vi "RSA306 hi with FFTsub3.vi"() -> ()   [LabVIEW 2016]
doc: "This VI demonstrates a simple procedure for setting up a spectrum analyzer, running an acquisition, and retrieving and plotting the waveform data.\n\nString indicators Binary WF Data and Sgl Float WF Data are initialized to empty strings. Waveform Graph is initialized to 0 for 100000 locations (just an arbitrary number for demonstration purposes).\n\ntkrsa6100 Initialize.vi opens the VISA Resource Name from the information entered by the user. It also presets the instrument by default to the Spectrum measurement. On completion it passes dup VISA Resource Name and error out to the following drivers.\n\nThe next VI to execute is tkrsa6100 Config Frequency.vi. Numeric control Center Freq (MHz)(50) is passed to the VI to set the center frequency to the default 50MHz value. The Set/Read Freq Setting (Set) is not wired since it defaults to SET, which is what is desired in this case. This is the case for all the configuration VI's in the example.\n\nThe next VI to execute is tkrsa6100 Config Spectrum Settings.vi. Enumerated control Spectrum Settings (CENTER FREQUENCY) is passed a Frequency Span constant and numeric control Freq Span (MHz) (40) to set the span to 40MHz.\n\nNext the reference level is set using tkrsa6100 Config RF Input.vi. Enumerated control Input Setting (REFERENCE LEVEL) is passed a Reference Level constant and numeric control Ref Level (dBm)(0) to set the reference level to 0dBm.\n\nNext the acquisition mode is set to single acquisition using tkrsa6100 Config Acquisition.vi. No parameters are passed since the default setting of this VI sets the acquisition mode to single.\n\nA single acquisition is then performed using tkrsa6100 Run Single Acquisition.vi. This VI sends an INIT command followed by a *OPC? Query. When the acquisition is completed the instrument returns a 1 and the next vi executes.\n\nThe binary waveform data is then retrieved by tkrsa6100 Spectrum Msmt Results.vi. The last acquisition data is retrieved by passing constant GET LAST ACQUISITION RESULT to enumerated input Run Acquisition and/or Get Result (RUN ACQUISITION & GET RESULT). The binary data is converted to a comma separated list of single precision floating point numbers by passing constant YES to enumerated input Convert Resp String (NO). The number of display points (total number of data bytes/4) is passed to a Spectral Display property node to scale the x axis of the graph. The binary data string from output Measurement Response String is copied to string indicator Binary WF Data. The converted binary data from output Converted Sgl Float Response String is copied to string indicator Sgl Float WF Data.\n\nSgl Float WF Data is then converted to an array by function Spreadsheet String to Array using a comma as the data separator. The output array is then passed to waveform graph Spectral Display for viewing.\n\nThe VISA Resource Name is closed using tkrsa6100 Close.vi."
uses:
  <vilib>/Analysis/baseanly.llb/Mean (DBL).vi
  <vilib>/Analysis/NI_AALBase.lvlib
panel:
  out "Peak vs time":cluster{i32[], dbl[]}(graph)
  out "mean":dbl format="%0.2f"
  out "Amp in range":dbl[](array[numeric])
  out "Pts in range":dbl[](array[numeric])
  in  "Marker Freq stop":dbl
  out "fractional index or x":dbl
  in  "Marker Freq start":dbl
  in  "stop 2":bool
  in  "RSA Control Cluster":T1={"Center Freq (MHz)"=20.0, "Freq Span (MHz)"=20.0, "Ref Level (dBm)"=0.0, "# Points"=enum."801", "Analysis Length (ms)"=0.022, "Trigger Settings\n(TRIGGER SOURCE)"=enum."TRIGGER ON"} {"Analysis Length (ms)" step=1e-09; "Ref Level (dBm)" min=-170.0 max=50.0 step=0.1}
  out "Metrics:Total Data Size":u32
  out "Metrics:Size of Front Panel":u32
  out "Freq Out Cluster":T2
  out "cursor diff":dbl
  out "iteration":i32
  out "# of Pts Between Cursors":dbl
  out "Cursor 1 X":dbl
  out "Cursor 0 X":dbl
  out "I & Q full":cluster{dbl[], "I or Q Data Array":sgl[]}[](graph)
  out "# of Spectrum pts retrieved":i32
  in  "stop":bool=TRUE
  in  "beta":dbl format="%0.2f"
  in  "Use windowing":bool
  out "FFT out From RSA":cluster{dbl[], "FFT {X}":dbl[]}(graph)
  out "FFT^2 from I&Q":cluster{dbl[], "FFT {X}":dbl[]}(graph)={[72.99999907342773, 73.14432898943954, 73.28865890545134, 73.43298882146314, 73.57731873747494, 73.72164865348674, 73.86597856949854, 74.01030848551034, 74.15463840152213, 74.29896831753393, 74.44329823354573, 74.58762814955753, 74.73195806556933, 74.87628798158114, 75.02061789759293, 75.16494781360473, 75.30927772961653, 75.45360764562834, 75.59793756164012, 75.74226747765192, 75.88659739366372, 76.03092730967553, 76.17525722568732, 76.31958714169912, 76.46391705771092, 76.60824697372273, 76.75257688973453, 76.89690680574631, 77.04123672175811, 77.18556663776992, 77.32989655378172, 77.4742264697935, 77.6185563858053, 77.76288630181712, 77.90721621782892, 78.05154613384072, 78.1958760498525, 78.34020596586431, 78.48453588187611, 78.62886579788791, 78.7731957138997, 78.91752562991151, 79.06185554592331, 79.2061854619351, 79.35051537794689, 79.4948452939587, 79.6391752099705, 79.7835051259823, 79.9278350419941, 80.0721649580059, 80.2164948740177, 80.3608247900295, 80.5051547060413, 80.64948462205311, 80.7938145380649, 80.93814445407669, 81.08247437008849, 81.2268042861003, 81.37113420211209, 81.51546411812389, 81.65979403413569, 81.8041239501475, 81.94845386615928, 82.09278378217108, 82.23711369818288, 82.3814436141947, 82.5257735302065, 82.67010344621828, 82.81443336223008, 82.95876327824189, 83.10309319425369, 83.24742311026547, 83.39175302627727, 83.53608294228908, 83.68041285830088, 83.82474277431268, 83.96907269032447, 84.11340260633628, 84.25773252234808, 84.40206243835988, 84.54639235437166, 84.69072227038347, 84.83505218639527, 84.97938210240707, 85.12371201841886, 85.26804193443067, 85.41237185044247, 85.55670176645427, 85.70103168246607, 85.84536159847787, 85.98969151448966, 86.13402143050146, 86.27835134651326, 86.42268126252506, 86.56701117853686, 86.71134109454866, 86.85567101056046], "FFT {X}"=[2.273932630988823e-07, 1.1331146319928143e-07, 7.673719462960696e-08, 4.8490746468829755e-06, 1.6442867833395572e-06, 3.16436268703382e-06, 2.639540533574584e-06, 3.334839091433884e-06, 4.600463519168855e-07, 7.66410378536425e-06, 2.1359108019339082e-05, 3.163756375846005e-05, 1.7486392953015998e-06, 5.819774956187226e-05, 1.7641054577208325e-05, 1.6979948996099875e-05, 6.2693899532632095e-06, 2.3345502675972444e-06, 3.1376219779214914e-05, 2.03224790497132e-05, 1.615880551905034e-05, 1.0387525314792172e-05, 1.5288981152198085e-05, 8.951089675188266e-05, 5.220838568835042e-06, 3.951059482528036e-06, 2.2455332453227875e-05, 4.043265080177603e-05, 1.3603674976209462e-05, 1.4610779340262739e-05, 6.778155093094428e-06, 5.92310092221894e-05, 0.00012371060242161107, 4.2293965227730726e-05, 4.793949807803902e-06, 1.703774948817084e-05, 4.1046539738076146e-05, 1.0575250111078698e-05, 1.5838772387061695e-05, 5.963059605451412e-06, 8.322466613350297e-06, 4.241894423745356e-05, 2.5902944249513385e-05, 3.754440849478757e-06, 2.2684130780756104e-06, 1.4792708956558557e-06, 2.8052728218109083e-06, 9.519822607230608e-06, 2.5898912044999134e-07, 1.5674000233301835e-05, 1.3652167200969293e-06, 1.9463849822553144e-06, 3.654050359843304e-05, 1.1291499237591179e-05, 6.364356455835304e-06, 1.5162644733310776e-05, 2.498743892235212e-05, 2.59215466998731e-05, 2.5356348978855883e-05, 3.372928674635838e-05, 3.2302722433788863e-06, 6.456706467716242e-06, 1.458542775043343e-05, 6.265393201875059e-06, 1.0526946272506417e-05, 1.3629572719674517e-05, 5.08190028344042e-06, 8.753167304918669e-06, 1.0618177493791915e-05, 4.256799122932561e-05, 6.634457042403187e-06, 1.2110046839534622e-05, 3.4087842403903063e-06, 6.274698806587281e-06, 1.7395492102973268e-05, 6.128606933081257e-05, 8.034267247831298e-05, 2.2934113274395202e-05, 3.215895946795535e-05, 1.0317162977800269e-06, 2.8731735651279777e-07, 2.8598897809844725e-05, 1.773915488316907e-06, 2.4559181515814637e-05, 6.51682013725626e-05, 1.3429668418120791e-05, 1.5195877753597404e-05, 7.288765358591678e-06, 1.8987776629762155e-05, 2.3445741553836735e-05, 2.5513476948437664e-06, 7.888513041438307e-07, 1.3567788998363706e-06, 2.0658168696090098e-06, 5.785587479331871e-07, 2.8232882934250476e-07, 2.6643643406101695e-07]}
  out "FreqStep":dbl
  out "I & Q  partial":cluster{dbl[], sgl[]}[](graph)
  out "# I or Q Pts":i32
  in  "VISA Resource Name":refnum<visa-resource-name>="TCPIP0::127.0.0.1::inst0::INSTR"
  out "Sgl Float WF Data":string
  out "Binary WF Data":string
  out "Spectral Display":dbl[](graph)=[-100.550338745117, -100.865898132324, -100.055114746094, -100.513687133789, -98.912384033203, -101.86759185791, -99.886054992676, -98.280754089355, -99.356986999512, -99.41291809082, -100.67155456543, -100.569961547852, -101.467147827148, -99.184501647949, -101.941261291504, -100.212478637695, -101.129829406738, -100.52604675293, -100.7939453125, -100.198677062988, -100.002563476562, -101.958740234375, -99.303619384766, -98.484771728516, -100.796211242676, -101.325035095215, -101.804656982422, -100.850593566895, -101.298637390137, -99.770805358887, -98.808280944824, -101.318023681641, -99.57886505127, -100.508224487305, -100.616767883301, -100.600654602051, -99.123565673828, -101.568901062012, -98.457931518555, -99.805709838867, -99.298568725586, -102.226028442383, -100.700386047363, -99.445762634277, -100.692687988281, -100.283546447754, -101.525848388672, -101.59400177002, -100.571098327637, -100.408309936523, -101.573852539062, -100.876373291016, -99.473991394043, -98.885787963867, -99.478179931641, -99.414611816406, -100.745628356934, -100.405769348145, -100.550086975098, -101.737022399902, -100.464469909668, -102.024978637695, -100.643768310547, -100.495559692383, -100.85823059082, -100.459129333496, -100.412284851074, -99.047401428223, -100.545104980469, -100.606239318848, -100.008010864258, -101.58097076416, -99.201164245605, -100.060760498047, -99.007080078125, -98.575668334961, -100.801124572754, -101.846046447754, -100.409858703613, -99.658515930176, -87.074851989746, -101.954887390137, -101.25106048584, -100.35228729248, -100.468887329102, -100.489883422852, -100.308792114258, -99.900894165039, -100.278121948242, -99.058067321777, -99.013816833496, -100.399383544922, -101.039794921875, -98.751235961914, -101.476287841797, -100.809410095215, -101.54175567627, -100.014114379883, -98.903923034668, -100.957069396973, -100.160820007324, -100.303314208984, -101.395530700684, -101.13591003418, -100.250480651855, -100.815155029297, -101.235824584961, -100.353385925293, -100.524604797363, -101.694984436035, -100.57209777832, -100.20694732666, -100.339385986328, -100.5029296875, -102.065803527832, -100.840377807617, -101.361434936523, -102.486083984375, -99.822219848633, -99.708770751953, -100.815650939941, -99.921195983887, -99.004348754883, -101.069366455078, -100.102096557617, -101.359786987305, -100.169326782227, -100.855087280273, -100.436889648437, -99.430320739746, -102.201194763184, -98.398323059082, -100.264114379883, -101.190093994141, -97.551864624023, -99.804649353027, -100.999176025391, -102.163314819336, -99.233787536621, -101.160591125488, -102.859664916992, -100.933372497559, -99.543952941895, -101.640991210937, -100.737907409668, -100.88272857666, -99.914588928223, -100.99201965332, -99.82975769043, -99.958145141602, -100.332321166992, -99.202865600586, -98.971542358398, -101.199119567871, -100.002639770508, -100.379287719727, -102.733993530273, -101.047821044922, -101.062637329102, -100.490631103516, -99.570091247559, -100.822036743164, -99.495933532715, -99.691299438477, -101.119491577148, -99.969169616699, -101.370628356934, -101.276794433594, -100.304641723633, -97.739120483398, -99.724952697754, -98.052604675293, -101.780364990234, -99.872802734375, -101.446601867676, -100.011825561523, -100.626129150391, -100.016258239746, -100.463325500488, -100.814552307129, -98.368011474609, -101.450942993164, -98.984527587891, -99.13134765625, -101.283500671387, -101.268920898437, -99.028633117676, -99.825736999512, -99.720832824707, -101.301513671875, -101.047241210937, -100.3115234375, -100.123146057129, -99.407669067383, -99.631744384766, -100.10962677002, -100.001708984375, -102.515518188477, -98.70344543457, -100.51188659668, -98.830825805664, -99.284408569336, -100.024505615234, -98.385818481445, -100.892181396484, -99.685241699219, -98.992698669434, -99.39395904541, -100.281867980957, -99.531661987305, -100.906555175781, -99.699020385742, -100.121429443359, -98.757469177246, -99.419845581055, -97.976013183594, -101.205871582031, -100.501953125, -100.021583557129, -100.356979370117, -100.71753692627, -100.46329498291, -100.892501831055, -101.838409423828, -101.372383117676, -99.252029418945, -99.76936340332, -98.654335021973, -100.489685058594, -99.062408447266, -101.665840148926, -99.905433654785, -101.712501525879, -99.85466003418, -100.939422607422, -98.979385375977, -101.255149841309, -101.09969329834, -100.925674438477, -100.328742980957, -99.538612365723, -98.808433532715, -100.842529296875, -100.238067626953, -101.345428466797, -100.050537109375, -100.399284362793, -100.017051696777, -99.849670410156, -100.567657470703, -100.343772888184, -99.282569885254, -100.663917541504, -101.199584960937, -101.901153564453, -101.351409912109, -98.658866882324, -99.848770141602, -101.877182006836, -100.49617767334, -101.537330627441, -100.924682617187, -97.984771728516, -100.308158874512, -100.322402954102, -100.767883300781, -100.310073852539, -100.786071777344, -101.351623535156, -100.523536682129, -101.092514038086, -100.754669189453, -99.298774719238, -100.813056945801, -99.991065979004, -101.504623413086, -101.232765197754, -100.107154846191, -99.418594360352, -98.61107635498, -99.415710449219, -101.472129821777, -100.912246704102, -99.791061401367, -101.327758789062, -100.108337402344, -100.526657104492, -99.587135314941, -98.377944946289, -100.356819152832, -99.85327911377, -100.841262817383, -98.974731445312, -99.606948852539, -102.143646240234, -98.766189575195, -99.99284362793, -100.895263671875, -99.367050170898, -99.253242492676, -100.08667755127, -100.553131103516, -100.857391357422, -101.711227416992, -99.825546264648, -98.692436218262, -99.648223876953, -99.844596862793, -99.068862915039, -101.533081054687, -99.982055664062, -100.804931640625, -96.95915222168, -100.675964355469, -100.574676513672, -99.792411804199, -100.516044616699, -99.432067871094, -101.020401000977, -100.661483764648, -101.725570678711, -99.595375061035, -100.06787109375, -99.804389953613, -102.322189331055, -98.901550292969, -101.507293701172, -99.793487548828, -100.540351867676, -100.780242919922, -100.127319335937, -100.003524780273, -99.602500915527, -98.637382507324, -101.011360168457, -99.077499389648, -100.247482299805, -97.887725830078, -102.085151672363, -99.34139251709, -100.531723022461, -100.816795349121, -102.088920593262, -100.546455383301, -102.192306518555, -99.071624755859, -100.28343963623, -100.598419189453, -99.334259033203, -99.664779663086, -97.886917114258, -99.813995361328, -100.696228027344, -101.955505371094, -102.258979797363, -102.029754638672, -100.8662109375, -100.926208496094, -100.807052612305, -101.128890991211, -98.354034423828, -99.024314880371, -101.485443115234, -101.602096557617, -97.892822265625, -101.470703125, -98.830749511719, -100.045959472656, -100.344650268555, -101.595001220703, -97.871208190918, -101.413185119629, -100.882888793945, -98.795585632324, -101.501831054687, -100.533180236816, -101.440567016602, -99.224174499512, -99.32649230957, -100.897682189941, -99.851852416992, -99.728507995605, -99.662971496582, -98.721755981445, -101.032135009766, -100.706283569336, -100.466918945312, -99.798248291016, -100.419586181641, -100.837371826172, -101.374435424805, -100.814964294434, -99.004135131836, -101.148536682129, -100.68058013916, -100.756843566895, -100.15885925293, -99.221481323242, -99.54581451416, -100.453453063965, -100.57795715332, -101.148979187012, -100.433052062988, -101.978225708008, -99.846565246582, -100.104637145996, -100.098175048828, -102.141723632812, -101.605690002441, -99.873359680176, -101.258079528809, -101.42431640625, -99.871452331543, -102.639274597168, -100.601585388184, -101.972610473633, -101.68872833252, -100.650726318359, -100.978286743164, -100.009384155273, -99.023010253906, -102.653121948242, -100.426239013672, -100.945854187012, -100.945205688477, -101.281471252441, -99.653778076172, -101.798393249512, -101.911247253418, -99.407638549805, -100.486267089844, -100.227569580078, -100.53246307373, -100.187919616699, -100.094390869141, -100.00910949707, -99.580986022949, -101.552139282227, -99.501281738281, -100.229248046875, -100.41072845459, -99.136566162109, -100.057098388672, -99.654800415039, -101.470153808594, -100.272033691406, -102.090690612793, -100.150230407715, -100.233016967773, -99.821128845215, -101.96110534668, -100.44783782959, -100.379745483398, -100.564086914062, -100.66283416748, -100.941314697266, -99.063705444336, -101.046104431152, -101.203369140625, -101.31706237793, -99.69482421875, -99.850654602051, -100.772903442383, -100.658180236816, -100.794387817383, -101.259185791016, -99.263107299805, -102.132049560547, -101.211318969727, -101.490661621094, -100.15983581543, -100.298202514648, -100.612930297852, -100.09033203125, -97.22306060791, -99.894561767578, -101.341903686523, -99.349258422852, -100.165794372559, -101.825523376465, -99.893409729004, -100.450881958008, -100.050659179687, -101.527481079102, -101.331695556641, -100.468971252441, -101.455322265625, -99.166534423828, -99.911262512207, -101.425621032715, -100.859977722168, -100.757179260254, -101.168304443359, -99.792510986328, -99.813842773437, -100.985527038574, -100.48152923584, -101.116722106934, -100.52799987793, -102.19359588623, -98.876556396484, -101.040328979492, -102.055938720703, -101.163955688477, -99.716537475586, -100.167327880859, -100.142478942871, -101.779495239258, -100.689811706543, -98.207588195801, -100.404693603516, -100.201606750488, -100.779479980469, -99.916084289551, -99.407791137695, -100.122749328613, -101.812606811523, -101.024642944336, -102.179672241211, -100.940444946289, -100.357330322266, -100.155799865723, -99.45484161377, -100.356147766113, -99.973617553711, -99.72966003418, -100.918563842773, -99.232574462891, -100.032485961914, -100.875595092773, -101.141540527344, -102.283218383789, -101.503074645996, -102.207214355469, -101.424591064453, -99.745712280273, -101.473587036133, -100.337684631348, -102.04655456543, -101.569664001465, -100.722312927246, -101.008522033691, -100.684356689453, -101.044158935547, -100.232864379883, -100.195053100586, -100.292091369629, -102.663642883301, -98.514129638672, -100.355270385742, -100.902053833008, -100.774368286133, -99.509002685547, -101.305000305176, -99.386489868164, -99.192878723145, -99.583618164062, -98.280197143555, -101.662719726562, -101.981384277344, -99.561195373535, -101.218673706055, -101.522567749023, -100.710975646973, -99.873352050781, -100.043991088867, -100.786987304687, -100.88207244873, -101.670349121094, -101.070434570312, -102.330474853516, -101.139305114746, -100.553726196289, -101.080917358398, -100.014381408691, -100.74267578125, -101.376068115234, -99.508666992187, -100.402755737305, -101.458442687988, -99.817077636719, -99.497161865234, -99.722450256348, -101.075325012207, -101.166007995605, -101.071212768555, -99.873245239258, -100.388832092285, -101.41625213623, -100.525978088379, -100.986129760742, -99.89119720459, -100.209266662598, -101.846252441406, -100.338325500488, -99.660354614258, -99.571578979492, -102.133171081543, -100.463859558105, -100.218765258789, -100.48420715332, -98.158195495605, -101.068511962891, -100.645751953125, -100.28645324707, -100.960067749023, -102.125846862793, -99.240020751953, -100.359405517578, -100.035057067871, -100.114097595215, -101.306259155273, -99.285079956055, -100.391830444336, -99.01554107666, -100.258865356445, -98.728218078613, -100.905616760254, -101.235694885254, -99.772598266602, -102.705078125, -99.118644714355, -100.937576293945, -99.03776550293, -100.502166748047, -100.544166564941, -100.152221679687, -99.755935668945, -101.306137084961, -101.620468139648, -100.771682739258, -97.545074462891, -99.748275756836, -99.849456787109, -99.425132751465, -101.4501953125, -100.094604492187, -101.045394897461, -100.365760803223, -100.378326416016, -99.960372924805, -99.518020629883, -98.761451721191, -100.071517944336, -99.611015319824, -100.961112976074, -99.728225708008, -101.468490600586, -100.286552429199, -100.593269348145, -100.339752197266, -100.324165344238, -100.608863830566, -100.953826904297, -102.148063659668, -100.073135375977, -101.460403442383, -100.869049072266, -100.91569519043, -99.907760620117, -100.546600341797, -99.498947143555, -98.508110046387, -101.926765441895, -97.669898986816, -99.041915893555, -100.350219726562, -99.40697479248, -100.568992614746, -101.795227050781, -100.295150756836, -100.469528198242, -100.674736022949, -101.288589477539, -100.309440612793, -101.232971191406, -97.823684692383, -101.273803710937, -101.031936645508, -100.720474243164, -101.440956115723, -100.856010437012, -98.955215454102, -101.424751281738, -99.771881103516, -101.40625, -101.204063415527, -101.750625610352, -100.588256835937, -102.470924377441, -101.291969299316, -101.423835754395, -98.857757568359, -102.00910949707, -100.523918151855, -100.347198486328, -100.93798828125, -101.508415222168, -100.711967468262, -99.973365783691, -99.873085021973, -100.742347717285, -100.09001159668, -100.524185180664, -101.417045593262, -101.220520019531, -102.689018249512, -102.225723266602, -101.284866333008, -100.547622680664, -101.23991394043, -102.037322998047, -100.880744934082, -100.685493469238, -100.668258666992, -100.301788330078, -99.016708374023, -102.30345916748, -99.447540283203, -100.94401550293, -86.783302307129, -100.292877197266, -101.487869262695, -100.213653564453, -102.028007507324, -98.812118530273, -100.086151123047, -101.277923583984, -101.078903198242, -100.103454589844, -98.755073547363, -101.702529907227, -99.214538574219, -98.939552307129, -100.480224609375, -98.694679260254, -99.073760986328, -100.033782958984, -101.073501586914, -100.257873535156, -99.690689086914, -100.311141967773, -102.31135559082, -101.017456054687, -99.194183349609, -100.42781829834, -102.232551574707, -100.907676696777, -98.880035400391, -100.672286987305, -101.721580505371, -100.515151977539, -98.296730041504, -101.345634460449, -99.50260925293, -100.800369262695, -99.824249267578, -101.611465454102, -97.455688476562, -102.069770812988, -100.366958618164, -100.448394775391, -99.052459716797, -98.817855834961, -101.656845092773, -99.100914001465, -101.839515686035, -101.317642211914, -100.746368408203, -99.396423339844, -100.516006469727, -102.368705749512, -99.86840057373, -101.438186645508, -100.931861877441, -101.522415161133, -99.652969360352, -101.873107910156, -99.384582519531, -100.033912658691, -99.868743896484, -101.091194152832, -101.110298156738, -100.822662353516, -99.58659362793, -100.84928894043, -100.407035827637, -100.647857666016, -98.793746948242, -100.717239379883, -101.495048522949, -102.786880493164, -101.375053405762, -101.189392089844, -101.156097412109, -100.519378662109, -102.34831237793, -100.975868225098, -100.173492431641, -99.891387939453, -100.191482543945]
  out "error out":errorcluster {"code" format="%#.0f"}
  # "This VI has the setup parameters entered in a sub VI\nThe FFT calculation is done in a loop that allows the # of pts\nto FFT to be selected. Also windowing can be changed.\nWhen happy about the FFT then push the STOP button.\nVersion just h is this VI before the setup sub VI was used"
  # "RSA306 Acquire and Fetch"
  # "Spectrum"
  # "Needs trigger input to work"
  # "IQ vs Time"
  # "To Do: Use these cursers to graphically select \nthe time window to FFT"
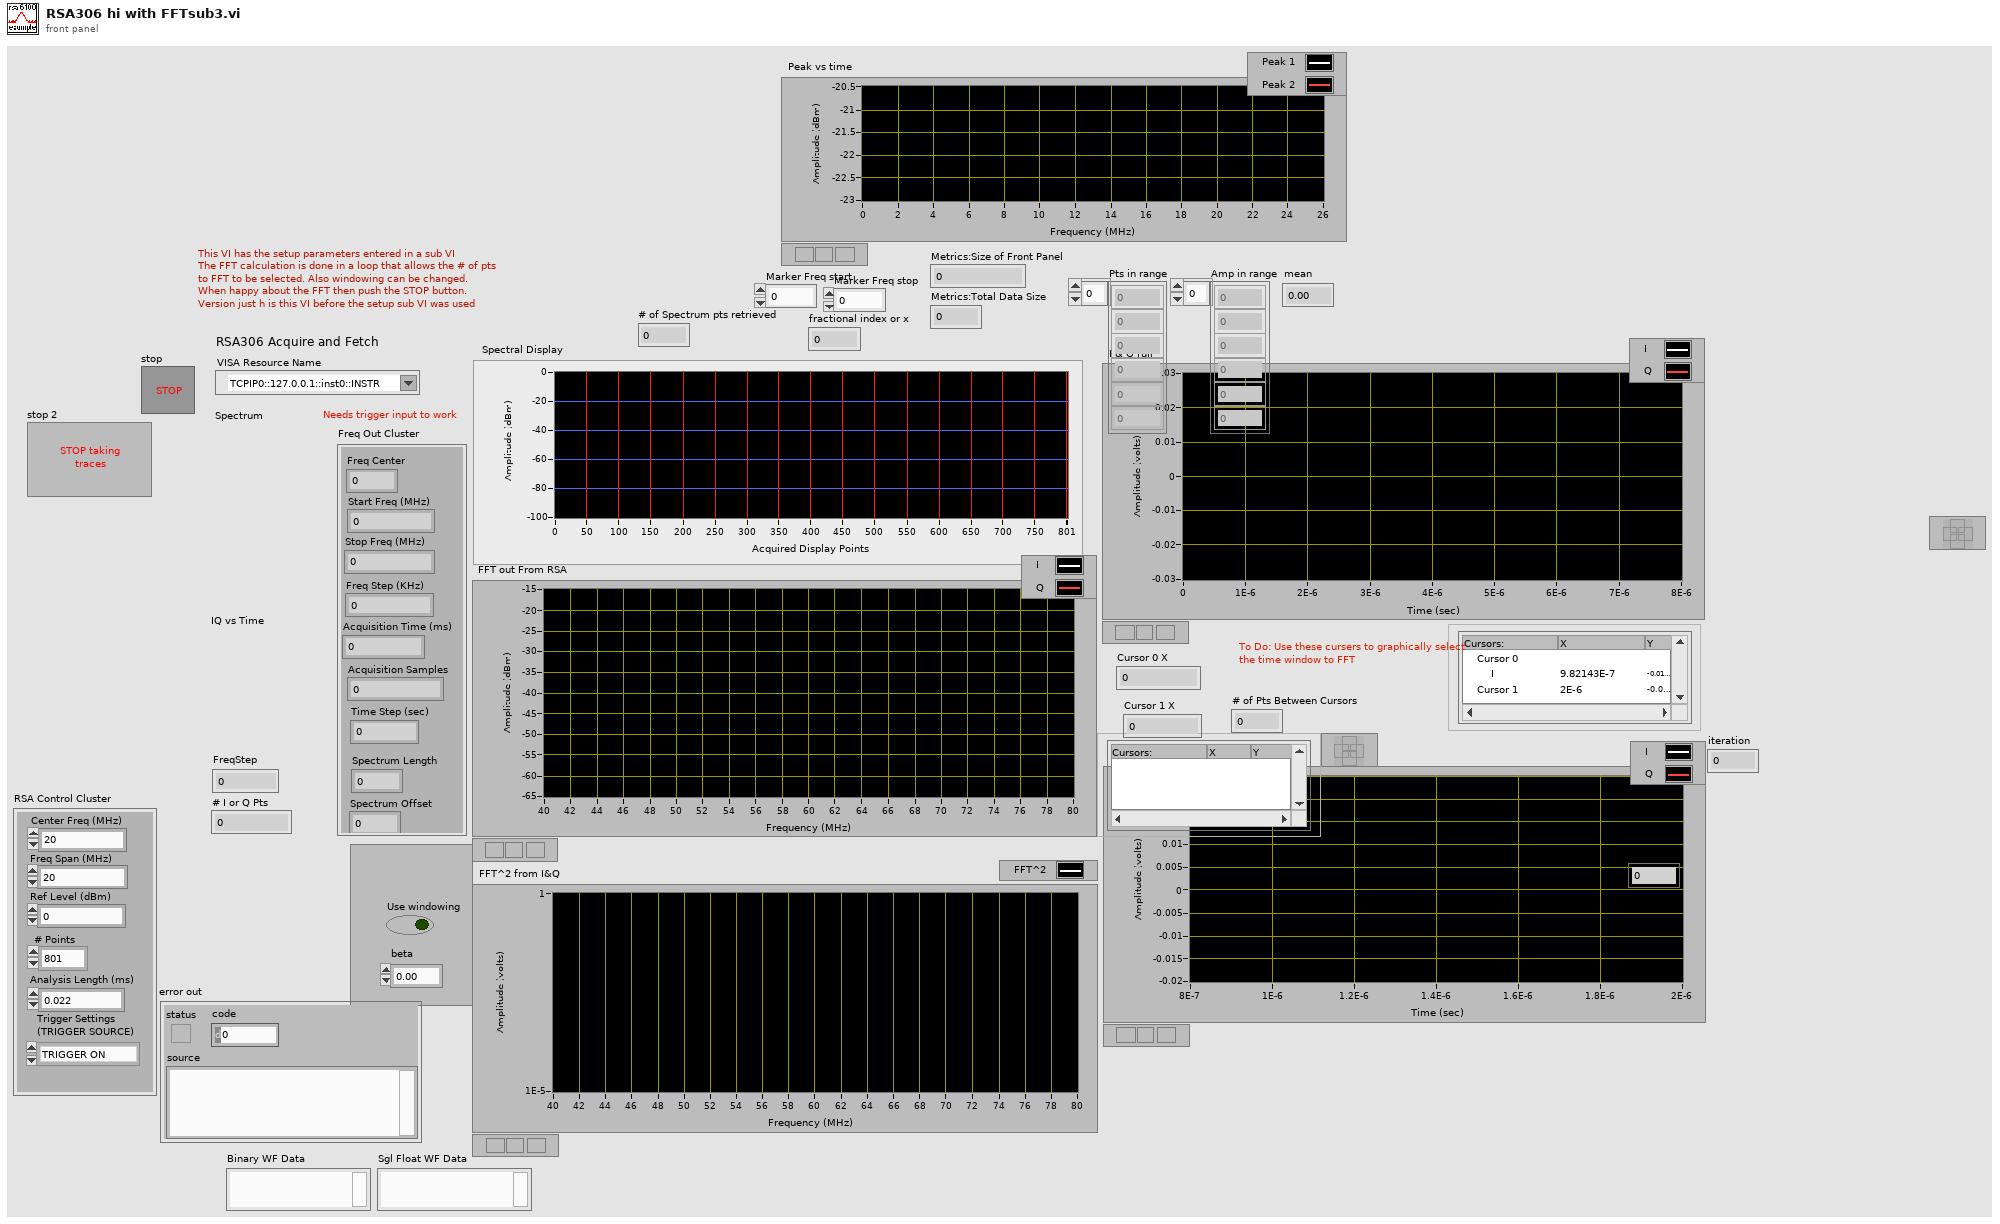
[diagram p1: front panel]
types:
  T1 = cluster{"Center Freq (MHz)":dbl, "Freq Span (MHz)":dbl, "Ref Level (dBm)":dbl, "# Points":enum16{"801", "2401", "4001", "8001", "10401", "16001", "32001", "64001"}, "Analysis Length (ms)":dbl, "Trigger Settings\n(TRIGGER SOURCE)":enum16{"TRIGGER SOURCE", "TRIGGER ON", "TRIGGER OFF", "TIME DELAY", "TIME POSITION", "TRIGGER EACH SEGMENT ON", "TRIGGER EACH SEGMENT OFF", "TRIGGER HOLDOFF ON", "TRIGGER HOLDOFF OFF", "TRIGGER HOLDOFF TIME", "FRONT EXT  LEVEL", "FRONT EXT IMPEDANCE", "FRONT EXT SLOPE", "REAR EXT SLOPE", "GATED TRIG2 (REAR) LOGIC", "FORCE TRIGGER (SET)"}}
  T2 = cluster{"Start Freq (MHz)":dbl, "Stop Freq (MHz)":dbl, "Freq Center":dbl, "Freq Step (KHz)":dbl, "Acquisition Time (ms)":dbl, "Acquisition Samples":dbl, "Time Step (sec)":dbl, "Spectrum Length":dbl, "Spectrum Offset":dbl}
  T3 = enum16{"RUN ACQUISITION  & GET RESULT", "GET LAST ACQUISITION RESULT"}
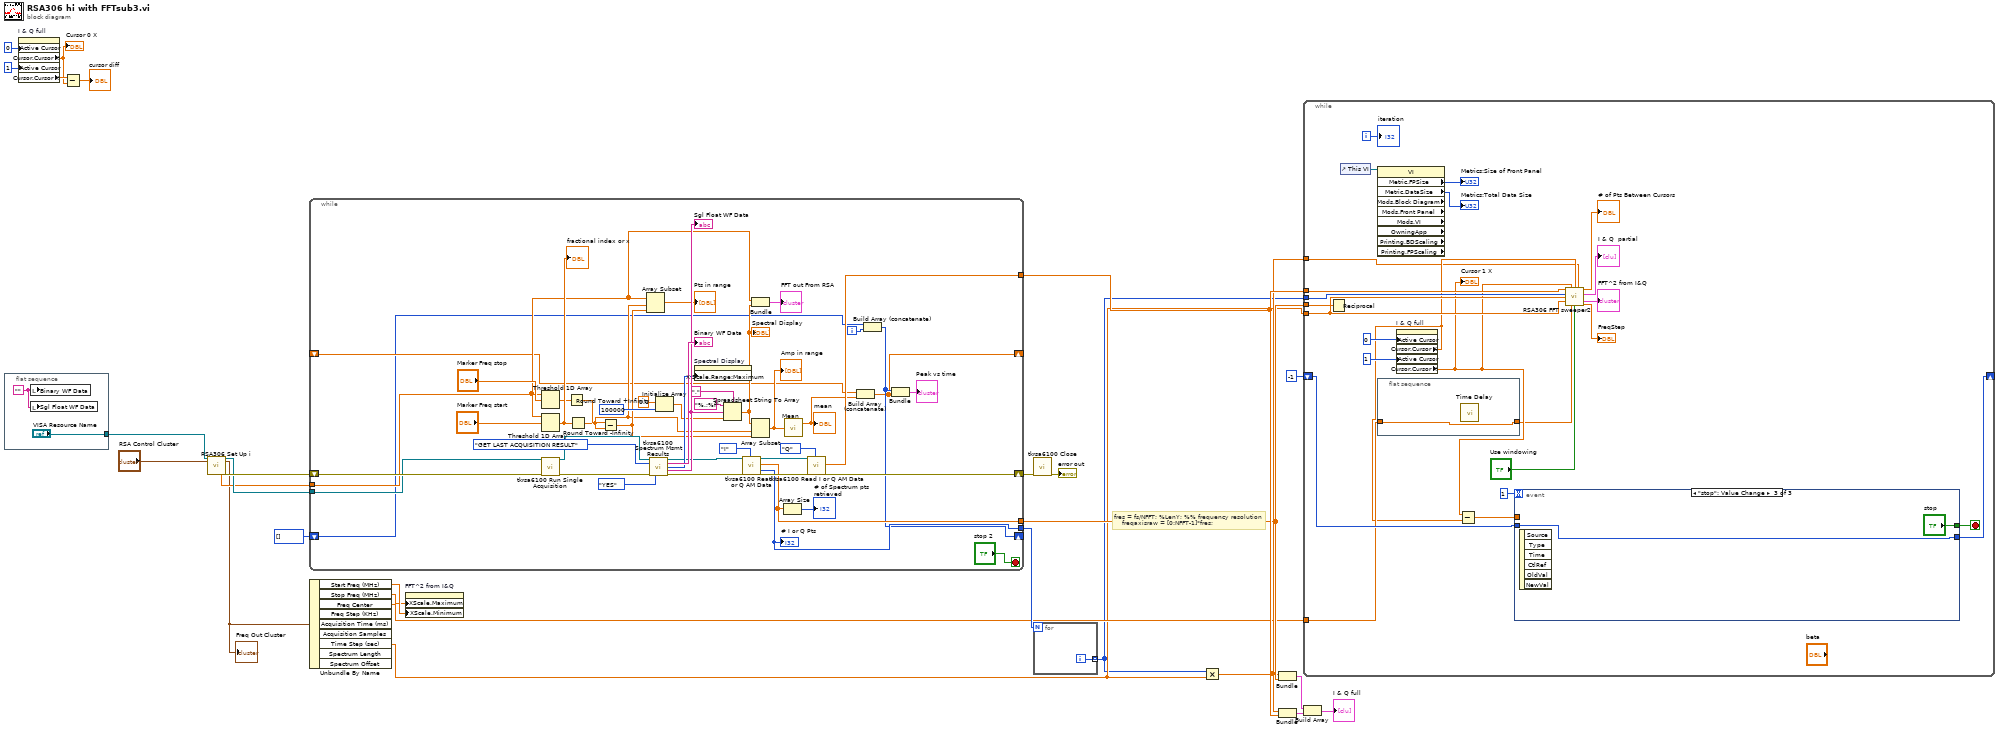
[diagram p0: block diagram]
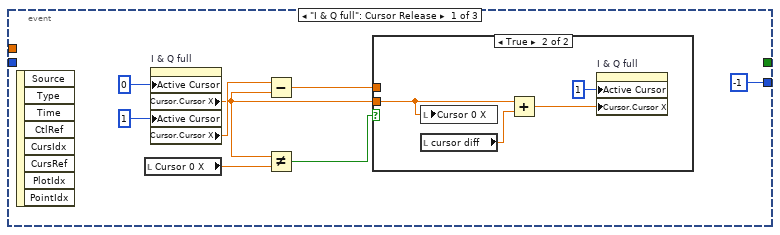
[diagram p2: hidden frame]
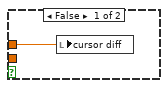
[diagram p3: hidden frame]
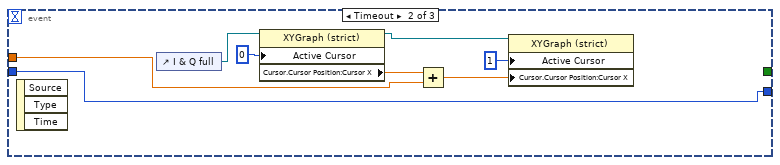
[diagram p4: hidden frame]
diagram:
  # "fres = fs/NFFT; %LenY; %% frequency resolution\n    freqaxisraw = [0:NFFT-1]*fres;"
  n1 = flat-sequence {
    tunnel: ["VISA Resource Name"] -> w22
    frame #0 {
      w29 = ""
      n2 = local write "Binary WF Data"(w29) -> ()
      n3 = local write "Sgl Float WF Data"(w29) -> ()
    }
  }
  n4 = property on="I & Q full" class="XYGraph (strict)"("Active Cursor"=u32 0, "Active Cursor"=u32 1) -> ("Cursor.Cursor X"=w9:dbl, "Cursor.Cursor X"=w11:dbl)  [unwired: 2 in, 2 out]
  "Cursor 0 X" <- w9
  n5 = Subtract(x=w11, y=w9) -> (x-y=→"cursor diff":dbl)
  n6 = call <instrlib>:"RSA306 Set Up i.vi"("VISA Resource Name"=w22, "RSA Control Cluster"="RSA Control Cluster") -> ("Freq Axis (MHz)"=w23:dbl[], "dup VISA Resource Name"=w24:refnum<visa-resource-name>, "Freq Out Cluster"=w8:T2, "error out"=w25:errorcluster)  [unwired: 14 in]
  "Freq Out Cluster" <- w8
  n7 = while {
    tunnel: w24 -> [w56]
    tunnel: w23 -> [w43]
    tunnel: [w51] -> w18
    tunnel: [w50] -> w17
    tunnel: [w49] -> w16
    shift-right: [w63] -> w26
    shift-left: w25 -> [w57]
    shift-right: [w32] -> _
    shift-left: i32[] [] -> [w35]
    shift-right: [w31] -> _
    shift-left: _ -> [w36]
    i -> [w33]
    stop <- "stop 2" stop-if-true
    n8 = Threshold 1D Array(2:"Marker Freq stop", 3:w43) -> (0:w44:dbl)  [unwired: 1 in]
    n9 = Threshold 1D Array(2:"Marker Freq start", 3:w43) -> (0:w45:dbl)  [unwired: 1 in]
    "fractional index or x" <- w45
    n10 = call <instrlib>:"tkrsa6100 Run Single Acquisition.vi"("VISA Resource Name"=w56, "error in (no error)"=w57) -> ("dup VISA Resource Name"=w59:refnum<visa-resource-name>, "error out"=w74:errorcluster)  [unwired: 12 out]
    n11 = Round Toward +Infinity(x=w44) -> (ceil(x): smallest int >= x=w42:dbl)
    n12 = Round Toward -Infinity(1:w45) -> (0:w39:dbl)
    n13 = Subtract(x=w42, y=w39) -> (x-y=w40:dbl)
    n14 = Array Subset(array=w43, index=w39, length=w40) -> (→"Pts in range":dbl[])
    n15 = call <instrlib>:"tkrsa6100 Spectrum Msmt Results.vi"("VISA Resource Name"=w59, "Run Acquisition and/or \nGet Result (RUN ACQUISITION & GET RESULT)"=T3."GET LAST ACQUISITION RESULT" ("Run Acquisition and/or \nGet Result (RUN ACQUISITION & GET RESULT)"), "error in (no error)"=w74, "Convert Resp\nString(NO)"=enum16{"NO", "YES"}."YES" ("Convert Resp\nString(NO)")) -> ("dup VISA Resource Name"=w58:refnum<visa-resource-name>, "Measurement\nResponse String"=→"Binary WF Data":string, "# Data Points"=w69:i32, "Converted Sgl Float\nResponse String"=w70:string, "error out"=w66:errorcluster)  [unwired: 3 in, 4 out]
    "Sgl Float WF Data" <- w70
    n16 = Initialize Array(0.0 ("element"), 100000 ("dimension size")) -> (w53:dbl[])
    n17 = property on="Spectral Display" class="WFGraph (strict)"("X Scale.Range:Maximum"=w69) -> ()  [unwired: 2 in, 2 out]
    n18 = Spreadsheet String To Array(delimiter (Tab)=",", format string="%.;%f", spreadsheet string=w70, array type (2D Dbl)=w53) -> (array=w38:dbl[])
    "Spectral Display" <- w38
    n19 = call <instrlib>:"tkrsa6100 Read I or Q AM Data.vi"("VISA Resource Name"=w58, "error in (no error)"=w66, "I or Q"=enum16{"I", "Q"}."I") -> ("dup VISA Resource Name"=w64:refnum<visa-resource-name>, "I or Q Data Array"=w49:sgl[], "# I or Q Pts"=w51:i32, "error out"=w65:errorcluster)  [unwired: 11 in, 2 out]
    "# I or Q Pts" <- w51
    n20 = Bundle("Freq Axis (MHz)"=w43, w38) -> (→"FFT out From RSA":cluster{"Freq Axis (MHz)":dbl[], dbl[]})  [unwired: 1 in]
    n21 = Array Subset(array=w38, index=w39, length=w40) -> (w37:dbl[])
    "Amp in range" <- w37
    n22 = Array Size(array=w49) -> (size(s)=→"# of Spectrum pts retrieved":i32)
    n23 = call-poly <vilib>:"Mean.vi"("X"=w37) -> ("mean"=w34:dbl)  [unwired: 1 out]
    "mean" <- w34
    n24 = call <instrlib>:"tkrsa6100 Read I or Q AM Data.vi"("VISA Resource Name"=w64, "error in (no error)"=w65, "I or Q"=enum16{"I", "Q"}."Q") -> ("I or Q Data Array"=w50:sgl[], "error out"=w63:errorcluster)  [unwired: 11 in, 4 out]
    n25 = Build Array (concatenate)(w36, w34) -> (w31:dbl[])
    n26 = Build Array (concatenate)(w35, w33) -> (w32:i32[])
    n27 = Bundle(w32, w31) -> (→"Peak vs time":cluster{i32[], dbl[]})  [unwired: 1 in]
  }
  n28 = Unbundle By Name(w8) -> ("Start Freq (MHz)"=w6:dbl, "Stop Freq (MHz)"=w5:dbl, "Freq Center"=w7:dbl, "Time Step (sec)"=w4:dbl)  [unwired: 5 out]
  n29 = property on="FFT^2 from I&Q" class="XYGraph (strict)"("XScale.Maximum"=w5, "XScale.Minimum"=w6) -> ()  [unwired: 2 in, 2 out]
  n30 = call <instrlib>:"tkrsa6100 Close.vi"("error in (no error)"=w26) -> ("error out"=→"error out":errorcluster)  [unwired: 1 in, 13 out]
  n31 = for {
    N: w18 -> [_]
    tunnel: [w75] -> w2 mode=indexing
    i -> [w75]
  }
  n32 = Multiply(x=w2, y=w4) -> (x*y=w15:dbl[])
  n33 = Bundle(w15, "I or Q Data Array"=w16) -> (w20:cluster{dbl[], "I or Q Data Array":sgl[]})  [unwired: 1 in]
  n34 = Bundle(w15, "I or Q Data Array"=w17) -> (w21:cluster{dbl[], "I or Q Data Array":sgl[]})  [unwired: 1 in]
  n35 = while {
    tunnel: w4 -> [w88]
    tunnel: w16 -> [w86]
    tunnel: w17 -> [w85]
    tunnel: w7 -> [w92]
    tunnel: w15 -> [w82]
    shift-right: [w97] -> _
    shift-left: -1 -> [w98]
    tunnel: w2 -> [w87]
    i -> [w94]
    stop <- w96 stop-if-true
    n36 = Reciprocal(x=w88) -> ()  [unwired: 1 out]
    n37 = control-ref of="This VI"() -> (w91:refnum<vi>)
    n38 = property class="VI" props=["Metric.FPSize", "Metric.DataSize", "Mods.Block Diagram", "Mods.Front Panel", "Mods.VI", "OwningApp", "Printing.BDScaling", "Printing.FPScaling"](reference=w91) -> ("Metric.FPSize"=→"Metrics:Size of Front Panel":u32, "Metric.DataSize"=→"Metrics:Total Data Size":u32)  [unwired: 1 in, 8 out]
    n39 = flat-sequence {
      tunnel: w92 -> [w101]
      tunnel: [w101] -> w81
      frame #0 {
        n40 = call "Time Delay"() -> ()  [unwired: 11 in, 1 out]
      }
    }
    n41 = property on="I & Q full" class="XYGraph (strict)"("Active Cursor"=u32 0, "Active Cursor"=u32 1) -> ("Cursor.Cursor X"=w84:dbl, "Cursor.Cursor X"=w83:dbl)  [unwired: 2 in, 2 out]
    "Cursor 1 X" <- w83
    n42 = Subtract(x=w83, y=w84) -> (x-y=w95:dbl)
    n43 = event shown="[2] \"stop\": Value Change" {
      selector: _ -> [_ _ _]
      dyn-events: _ -> [_ _ _]
      timeout: 1 -> [_ _ _]
      tunnel: [_ _ "stop"] -> w96
      tunnel: [-1 w122 w124] -> w97
      tunnel: w98 -> [_ w122 w124]
      tunnel: w95 -> [_ w115 _]
      event "I & Q full": Cursor Release {
        n44 = event-data() -> ()  [unwired: 1 in, 8 out]
        n45 = local read "Cursor 0 X"() -> (w106:dbl)
        n46 = property on="I & Q full" class="XYGraph (strict)"("Active Cursor"=u32 0, "Active Cursor"=u32 1) -> ("Cursor.Cursor X"=w103:dbl, "Cursor.Cursor X"=w104:dbl)  [unwired: 2 in, 2 out]
        n47 = Subtract(x=w104, y=w103) -> (x-y=w102:dbl)
        n48 = Not Equal?(x=w103, y=w106) -> (x != y?=w105:bool)
        n49 = case shown="True" w105 {
          tunnel: w103 -> [_ w111]
          tunnel: w102 -> [w110 _]
          frame False {
            n50 = local write "cursor diff"(w110) -> ()
          }
          frame True {
            n51 = local write "Cursor 0 X"(w111) -> ()
            n52 = local read "cursor diff"() -> (w113:dbl)
            n53 = Add(x=w111, y=w113) -> (x+y=w112:dbl)
            n54 = property on="I & Q full" class="XYGraph (strict)"("Active Cursor"=u32 1, "Cursor.Cursor X"=w112) -> ()  [unwired: 2 in, 2 out]
          }
        }
      }
      event Timeout {
        n55 = event-data() -> ()  [unwired: 1 in, 3 out]
        n56 = control-ref of="I & Q full"() -> (w116:refnum<vi>)
        n57 = property class="XYGraph (strict)"(reference=w116, "Active Cursor"=u32 0) -> (reference out=w119:refnum<vi>, "Cursor.Cursor Position:Cursor X"=w118:dbl)  [unwired: 1 in, 1 out]
        n58 = Add(x=w118, y=w115) -> (x+y=w117:dbl)
        n59 = property class="XYGraph (strict)"(reference=w119, "Active Cursor"=u32 1, "Cursor.Cursor Position:Cursor X"=w117) -> ()  [unwired: 1 in, 2 out]
      }
      event "stop": Value Change {
        n60 = event-data() -> ()  [unwired: 1 in, 6 out]
      }
    }
    n61 = call "RSA306 FFT sweeper2.vi"("Q Array"=w85, "2nd Cursor X"=w83, "1st Cursor X"=w84, "Time Array"=w82, "1toN Array"=w87, "I Array"=w86, "time step(sec)"=w88, "Freq Center"=w81, "Use windowing"="Use windowing") -> ("# of Pts Between cursors"=→"# of Pts Between Cursors":dbl, "I & Q  partial"=→"I & Q  partial":cluster{dbl[], sgl[]}[], "FFT^2 from partial"=→"FFT^2 from I&Q":cluster{dbl[], dbl[]}, "FreqStep"=→"FreqStep":dbl)  [unwired: 2 in, 1 out]
    "iteration" <- w94
  }
  n62 = Build Array(w20, w21) -> (→"I & Q full":cluster{dbl[], "I or Q Data Array":sgl[]}[])
